vi "Wait For LACK OF Front Panel Activity.vi"(0 "front panel (this VI's panel)":refnum<vi>, 1 "timeout (ms)":i32=1000) -> (8 "milliseccond timer value":u32)   [LabVIEW 2013]
doc: "Pauses the execution of the calling VI block diagram, until the function detects A LACK OF front panel activity, for the specified delay time, in the front panel being monitored."
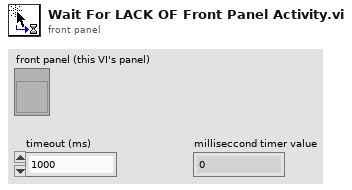
[diagram p1: front panel]
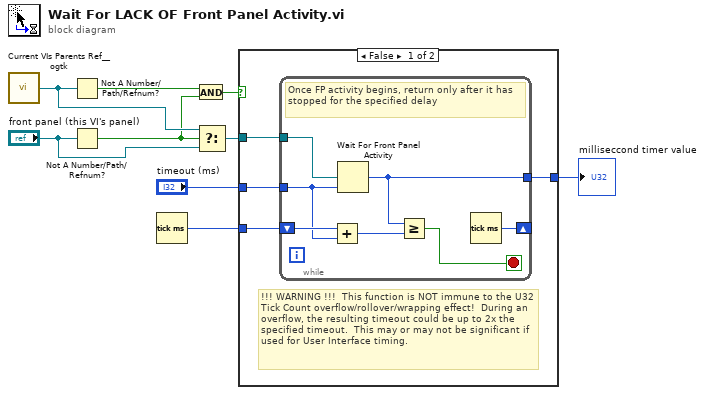
[diagram p0: block diagram]
diagram:
  n1 = call <userlib>:"Current VIs Parents Ref__ogtk.vi"() -> ("Calling VI's Reference"=w4:refnum<vi>)  [unwired: 2 in]
  n2 = Not A Number/Path/Refnum?(number/path/refnum=w4) -> (NaN/Path/Refnum?=w3:bool)
  n3 = Not A Number/Path/Refnum?(number/path/refnum="front panel (this VI's panel)") -> (NaN/Path/Refnum?=w2:bool)
  n4 = Tick Count (ms)() -> (millisecond timer value=w8:u32)
  n5 = And(x=w3, y=w2) -> (x .and. y?=w1:bool)
  n6 = Select(t=w4, s=w2, f="front panel (this VI's panel)") -> (s? t:f=w6:refnum<vi>)
  n7 = case shown="False" w1 {
    tunnel: "timeout (ms)" -> [w13 _]
    tunnel: w8 -> [w12 w21]
    tunnel: [w11 w21] -> w7
    tunnel: w6 -> [w10 _]
    frame False {
      # "!!! WARNING !!!  This function is NOT immune to the U32 Tick Count overflow/rollover/wrapping effect!  During an overflow, the resulting timeout could be up to 2x the specified timeout.  This may or may not be significant if used for User Interface timing."
      n8 = while {
        tunnel: w13 -> [w19]
        shift-right: [w17] -> _
        shift-left: w12 -> [w20]
        tunnel: [w16] -> w11
        tunnel: w10 -> [w14]
        stop <- w15 stop-if-true
        # "Once FP activity begins, return only after it has stopped for the specified delay"
        n9 = Add(x=w20, y=w19) -> (x+y=w18:u32)
        n10 = Wait For Front Panel Activity(1:w19, 2:w14) -> (0:w16:u32)  [unwired: 1 in]
        n11 = Greater Or Equal?(x=w16, y=w18) -> (x >= y?=w15:bool)
        n12 = Tick Count (ms)() -> (millisecond timer value=w17:u32)
      }
    }
    frame True {
      # "neither reference is valid"
    }
  }
  "milliseccond timer value" <- w7
